vi "Red_Light_Checker.vi"() -> ()   [LabVIEW 2015]
uses:
  SystemUtil/MotorStates.ctl
  Coll_Focus/GSP_COLL_Global.vi
  Slit/GSP_SLIT_Global.vi
  GSCS Scripting/Utils/GSP_Wavelength_Global.vi
  Grating_Translation/GSP_GT_Global.vi
  Cam_Focus/GSP_CF_Global.vi
  Primary Filter/GSP_F1_Global.vi
  Secondary Filter/GSP_F2_Global.vi
panel:
  out "Status":string
  in  "Clear Error":bool
  out "Response Error":errorcluster
  in  "Reset Motor":bool
  in  "Poll":bool
  in  "Select Motor:":u16(ring) items=["Collimator Focus"=40, "Camera Focus"=46, "Camera Angle"=45, "Grating Angle"=43, "Grating Translation"=44, "Secondary Filter"=48, "Primary Filter"=47, "Slit Translation"=42, "Slit Rotation"=41]
  in  "stop":bool
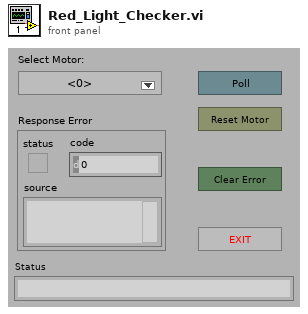
[diagram p1: front panel]
types:
  T1 = typedef "MotorStates.ctl" = enum16{"Ready", "Moving", "Uninitialized", "Error"}
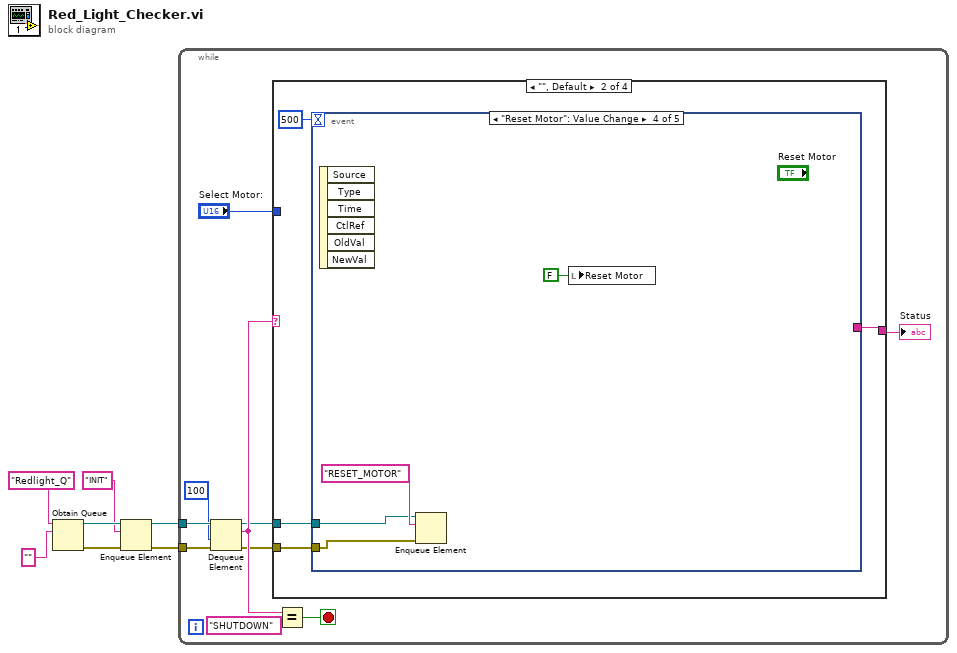
[diagram p0: block diagram]
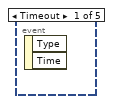
[diagram p3: hidden frame]
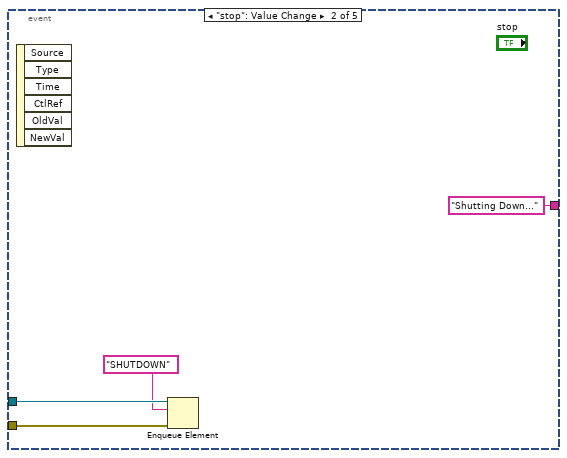
[diagram p4: hidden frame]
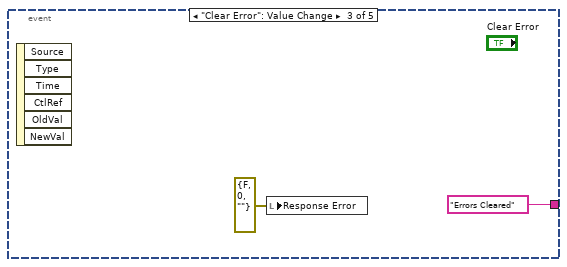
[diagram p5: hidden frame]
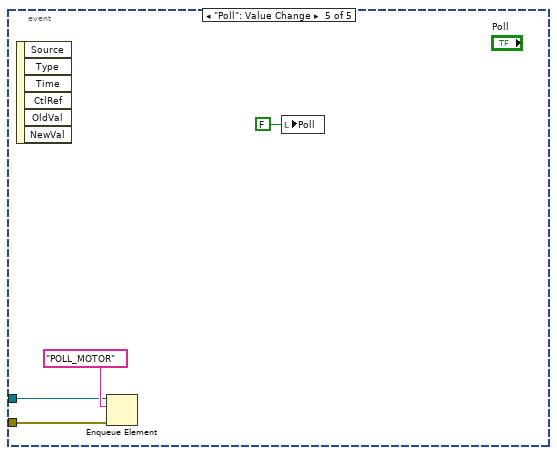
[diagram p6: hidden frame]
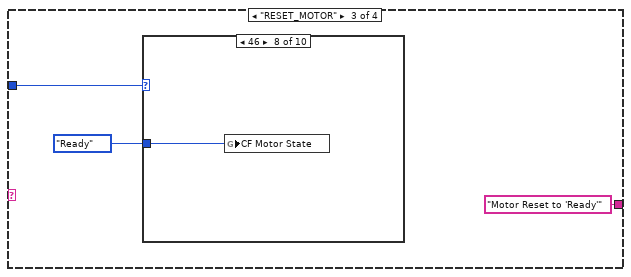
[diagram p7: hidden frame]
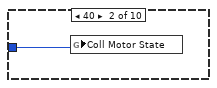
[diagram p9: hidden frame]
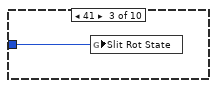
[diagram p10: hidden frame]
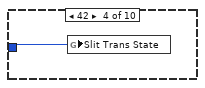
[diagram p11: hidden frame]
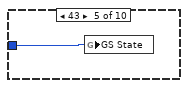
[diagram p12: hidden frame]
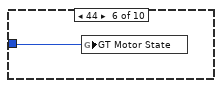
[diagram p13: hidden frame]
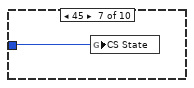
[diagram p14: hidden frame]
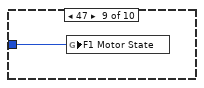
[diagram p15: hidden frame]
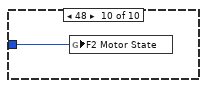
[diagram p16: hidden frame]
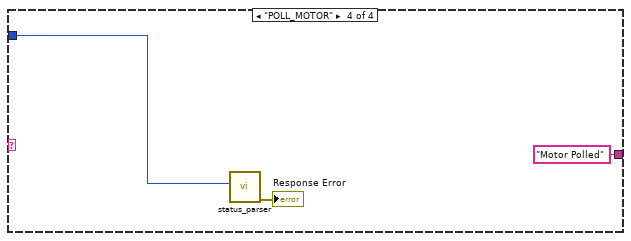
[diagram p17: hidden frame]
diagram:
  n1 = Obtain Queue(name (unnamed)="Redlight_Q", element data type="" ("y")) -> (queue out=w6:refnum<queue>, error out=w7:errorcluster)  [unwired: 3 in, 1 out]
  n2 = Enqueue Element(queue=w6, element="INIT", error in (no error)=w7) -> (queue out=w5:refnum<queue>, error out=w4:errorcluster)  [unwired: 1 in, 1 out]
  n3 = while {
    tunnel: w5 -> [w17]
    tunnel: w4 -> [w16]
    stop <- w14 stop-if-true
    n4 = Dequeue Element(queue=w17, timeout in ms (-1)=100, error in (no error)=w16) -> (queue out=w12:refnum<queue>, element=w13:string, error out=w11:errorcluster)  [unwired: 1 out]
    n5 = case shown="\"\", Default" w13 {
      tunnel: w12 -> [_ w21 _ _]
      tunnel: w11 -> [_ w20 _ _]
      tunnel: "Select Motor:" -> [_ _ w38 w50]
      tunnel: [_ w19 "Motor Reset to 'Ready'" "Motor Polled"] -> w9
      frame "False" {
      }
      frame "", Default {
        n6 = event shown="[3] \"Reset Motor\": Value Change" {
          selector: _ -> [_ _ _ _ _]
          dyn-events: _ -> [_ _ _ _ _]
          timeout: 500 -> [_ _ _ _ _]
          tunnel: w21 -> [_ w25 _ w29 w34]
          tunnel: w20 -> [_ w24 _ w28 w33]
          tunnel: [_ "Shutting Down..." "Errors Cleared" _ _] -> w19
          event Timeout {
            n7 = event-data() -> ()  [unwired: 1 in, 2 out]
          }
          event "stop": Value Change {
            n8 = event-data() -> ()  [unwired: 1 in, 6 out]
            n9 = Enqueue Element(queue=w25, element="SHUTDOWN", error in (no error)=w24) -> ()  [unwired: 1 in, 3 out]
          }
          event "Clear Error": Value Change {
            n10 = event-data() -> ()  [unwired: 1 in, 6 out]
            n11 = local write "Response Error"(errorcluster {"status"=FALSE, "code"=0, "source"=""} ("Response Error")) -> ()
          }
          event "Reset Motor": Value Change {
            n12 = event-data() -> ()  [unwired: 1 in, 6 out]
            n13 = Enqueue Element(queue=w29, element="RESET_MOTOR", error in (no error)=w28) -> ()  [unwired: 1 in, 3 out]
            n14 = local write "Reset Motor"(FALSE ("Reset Motor")) -> ()
          }
          event "Poll": Value Change {
            n15 = event-data() -> ()  [unwired: 1 in, 6 out]
            n16 = Enqueue Element(queue=w34, element="POLL_MOTOR", error in (no error)=w33) -> ()  [unwired: 1 in, 3 out]
            n17 = local write "Poll"(FALSE ("Poll")) -> ()
          }
        }
      }
      frame "RESET_MOTOR" {
        n18 = case shown="46" w38 {
          tunnel: MotorStates."Ready" ("CF Motor State") -> [_ w39 w40 w41 w42 w43 w44 w45 w46 w47]
          frame 0, Default {
          }
          frame 40 {
            n19 = global write "GSP_COLL_Global.vi" "Coll Motor State"(w39) -> ()
          }
          frame 41 {
            n20 = global write "GSP_SLIT_Global.vi" "Slit Rot State"(w40) -> ()
          }
          frame 42 {
            n21 = global write "GSP_SLIT_Global.vi" "Slit Trans State"(w41) -> ()
          }
          frame 43 {
            n22 = global write "GSP_Wavelength_Global.vi" "GS State"(w42) -> ()
          }
          frame 44 {
            n23 = global write "GSP_GT_Global.vi" "GT Motor State"(w43) -> ()
          }
          frame 45 {
            n24 = global write "GSP_Wavelength_Global.vi" "CS State"(w44) -> ()
          }
          frame 46 {
            n25 = global write "GSP_CF_Global.vi" "CF Motor State"(w45) -> ()
          }
          frame 47 {
            n26 = global write "GSP_F1_Global.vi" "F1 Motor State"(w46) -> ()
          }
          frame 48 {
            n27 = global write "GSP_F2_Global.vi" "F2 Motor State"(w47) -> ()
          }
        }
      }
      frame "POLL_MOTOR" {
        n28 = call "status_parser.vi"("Motor #"=w50) -> ("error out"=→"Response Error":errorcluster)  [unwired: 4 in, 2 out]
      }
    }
    "Status" <- w9
    n29 = Equal?(x=w13, y="SHUTDOWN") -> (x = y?=w14:bool)
  }
